vi "sio SetReadTimeouts.vi"(9 "字符间超时":u32, 10 "帧间超时":u32, 11 "port":i32) -> (0 "Status":i32, 3 "port":i32)   [LabVIEW 2015, in "PCOMM.lvlib"]
doc: "int WINAPI sio_SetTimeouts(int port, DWORD TotalTimeouts，DWORD IntervalTimeouts);\nTotalTimeouts：帧间超时间隔，单位是ms\nIntervalTimeouts：字符间超时间隔，单位是ms"
uses:
  PCOMM.lvlib
  PCOMM.DLL
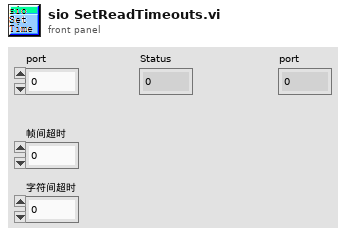
[diagram p1: front panel]
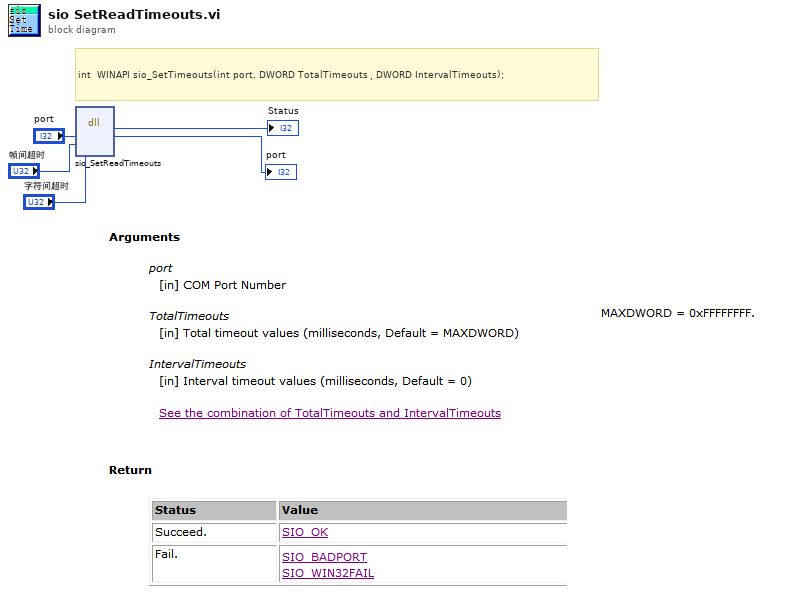
[diagram p0: block diagram]
diagram:
  # "int  WINAPI sio_SetTimeouts(int port, DWORD TotalTimeouts，DWORD IntervalTimeouts);"
  n1 = dll-call lib="PTH2^abs EDesktopLabview串口助手串口助手2.0Ing10_v3.2.0SubVIpcomm库PCOMM.*" fn="sio_SetReadTimeouts"("port"="port", "TotalTimeouts"="帧间超时", "IntervalTimeouts"="字符间超时") -> ("Status"=→"Status":i32, "port"=→"port":i32)  [unwired: 5 in, 2 out]
